vi "UART Open.vi"(8 "error in (no error)":errorcluster, 9 "Timeout (3s)":i32=3, 10 "Baud (115200)":i32=115200, 11 "Serial Port":i32) -> (0 "error out":errorcluster, 3 "Success?":bool)   [LabVIEW 2013]
uses:
  filter wheel/Libraries/uart_library.dll
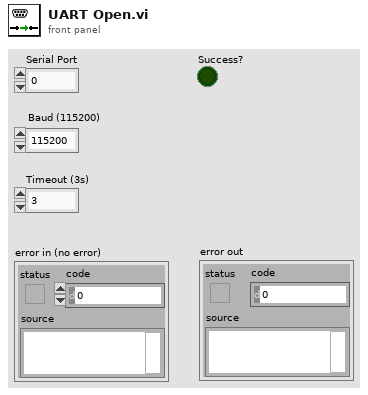
[diagram p1: front panel]
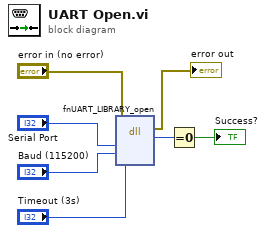
[diagram p0: block diagram]
diagram:
  n1 = dll-call lib="C:/Users/spim/Documents/Labview programs/2014_05_28 SPIM controller mathscript two colour/filter wheel/Libraries/uart_library.dll" fn="fnUART_LIBRARY_open"(error in="error in (no error)", "nPort"="Serial Port", "nBaud"="Baud (115200)", "Time"="Timeout (3s)") -> (error out=→"error out":errorcluster, "return type"=w5:i32)  [unwired: 5 in, 1 out]
  n2 = Equal To 0?(x=w5) -> (x = 0?=→"Success?":bool)
